vi "channel class to assembly type.vi"(11 "channel classification":T1) -> (3 "assembly types":T2)   [LabVIEW 2013, in "EIP Tags Channel.lvclass"]
uses:
  EIP Tags Channel.lvclass
  configuration/assembly type.ctl
  <vilib>/NI/Tag Bus Module Framework/channel/channel classification.ctl
  configuration/EIP Tags Configuration.lvclass
  <vilib>/NI/Tag Bus Module Framework/channel/TBM channel.lvclass
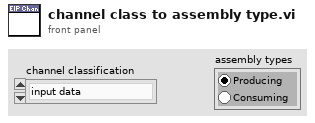
[diagram p1: front panel]
types:
  T1 = typedef "TBM channel.lvclass/channel classification.ctl" = enum16{"input data", "output data", "processing parameter", "processing result"}
  T2 = typedef "EIP Tags Configuration.lvclass/assembly type.ctl" = enum32{"Producing", "Consuming"}
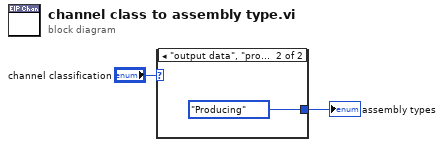
[diagram p0: block diagram]
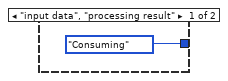
[diagram p2: hidden frame]
diagram:
  n1 = case shown="\"output data\", \"processing parameter\"" "channel classification" {
    tunnel: [assembly_type."Consuming" ("permissions") assembly_type."Producing" ("permissions")] -> w2
    frame "input data", "processing result" {
    }
    frame "output data", "processing parameter" {
    }
  }
  "assembly types" <- w2
